vi "導覽&溫度濕度_8月5號.vi"() -> ()   [LabVIEW 2019]
uses:
  Program Files (x86)/National Instruments/LabVIEW 2019/vi.lib/LabVIEW Interface for Arduino/Firmware/LIFA_Base/dht11/DHTXX.lvlib
  <vilib>/LabVIEW Interface for Arduino/LabVIEW Interface for Arduino.lvlib
panel:
  out "?":dbl
  out "濕度(%)":dbl(slide) scale=0.0..100.0
  out "?":dbl
  out "溫度(攝氏)":dbl(knob) scale=0.0..50.0
  in  "開始撥放(影片撥放時，其他作用暫時停用)":bool
  in  "Path":path
  in  "WindowsMediaPlayer":refnum<k7>(container)
  in  "檢測溫度濕度開關":bool
  in  "所有開關停止運作":bool
  out "運作中(燈亮)":bool
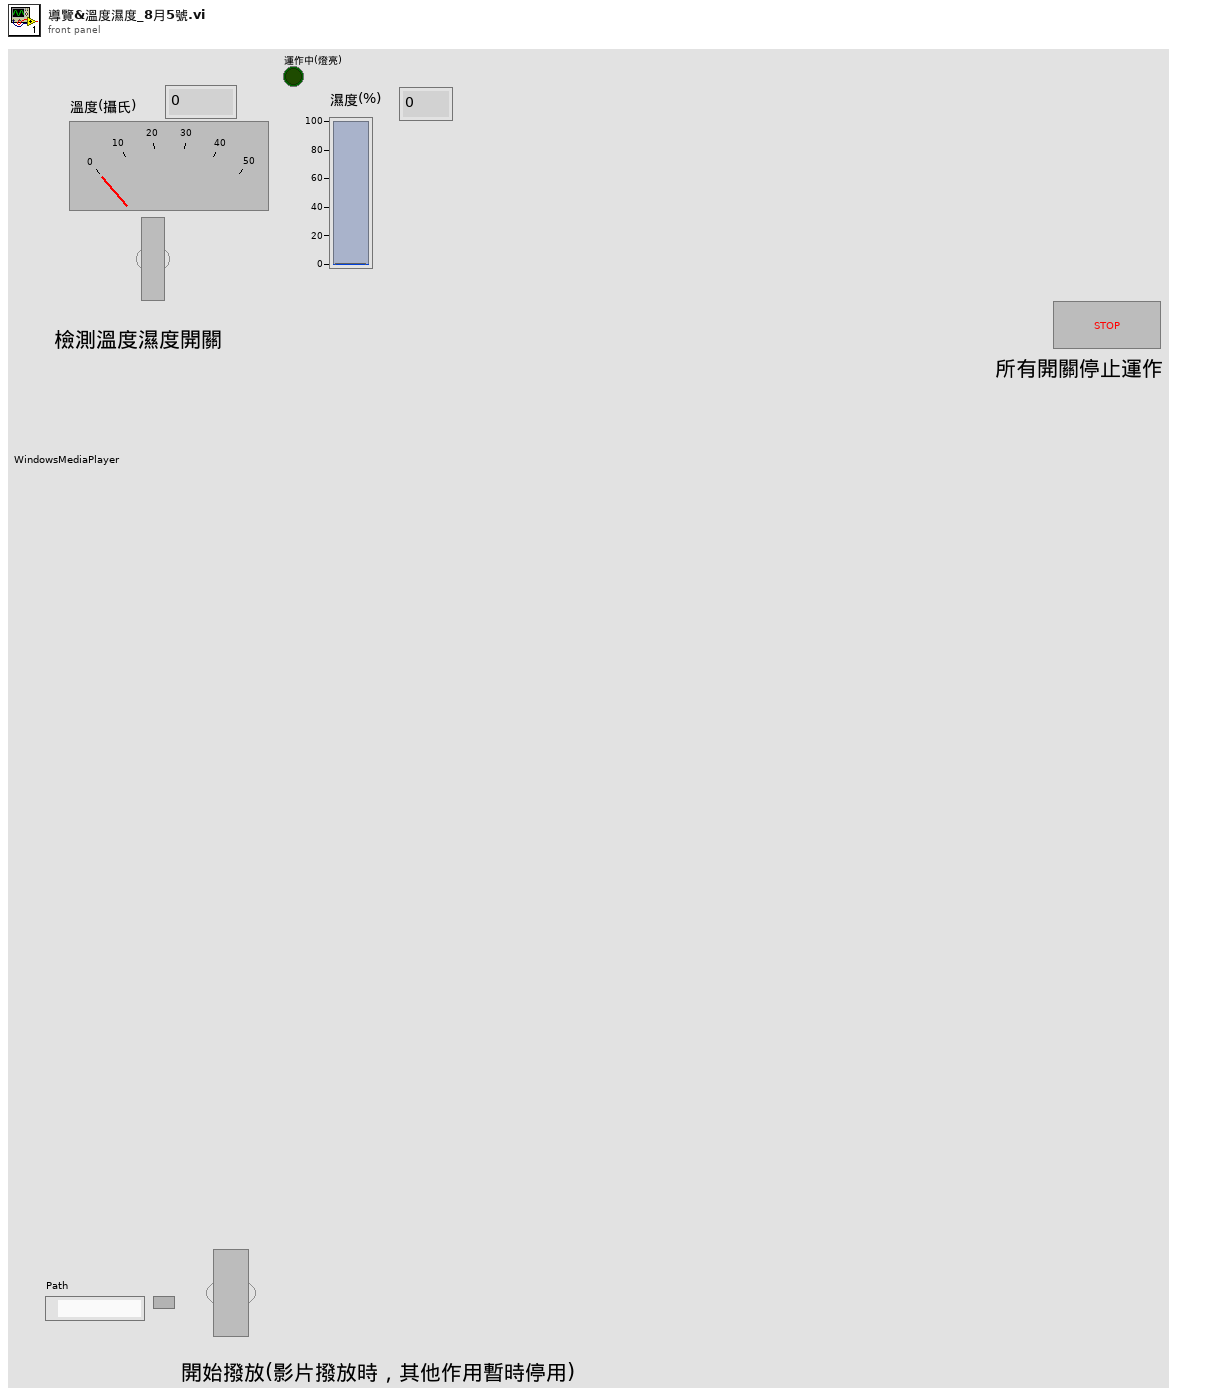
[diagram p1: front panel]
types:
  T1 = typedef "LabVIEW Interface for Arduino.lvlib/Arduino Resource.ctl" = cluster{"VISA resource":refnum<visa-resource-name>, "Board Type":T2, "Connection Type":enum8{"USB / Serial"}, "Bytes Per Packet (15)":u8}
  T2 = typedef "LabVIEW Interface for Arduino.lvlib/Board Type.ctl" = enum16{"Uno", "Dimuelanove w/Atmega 328", "Mega 2560"}
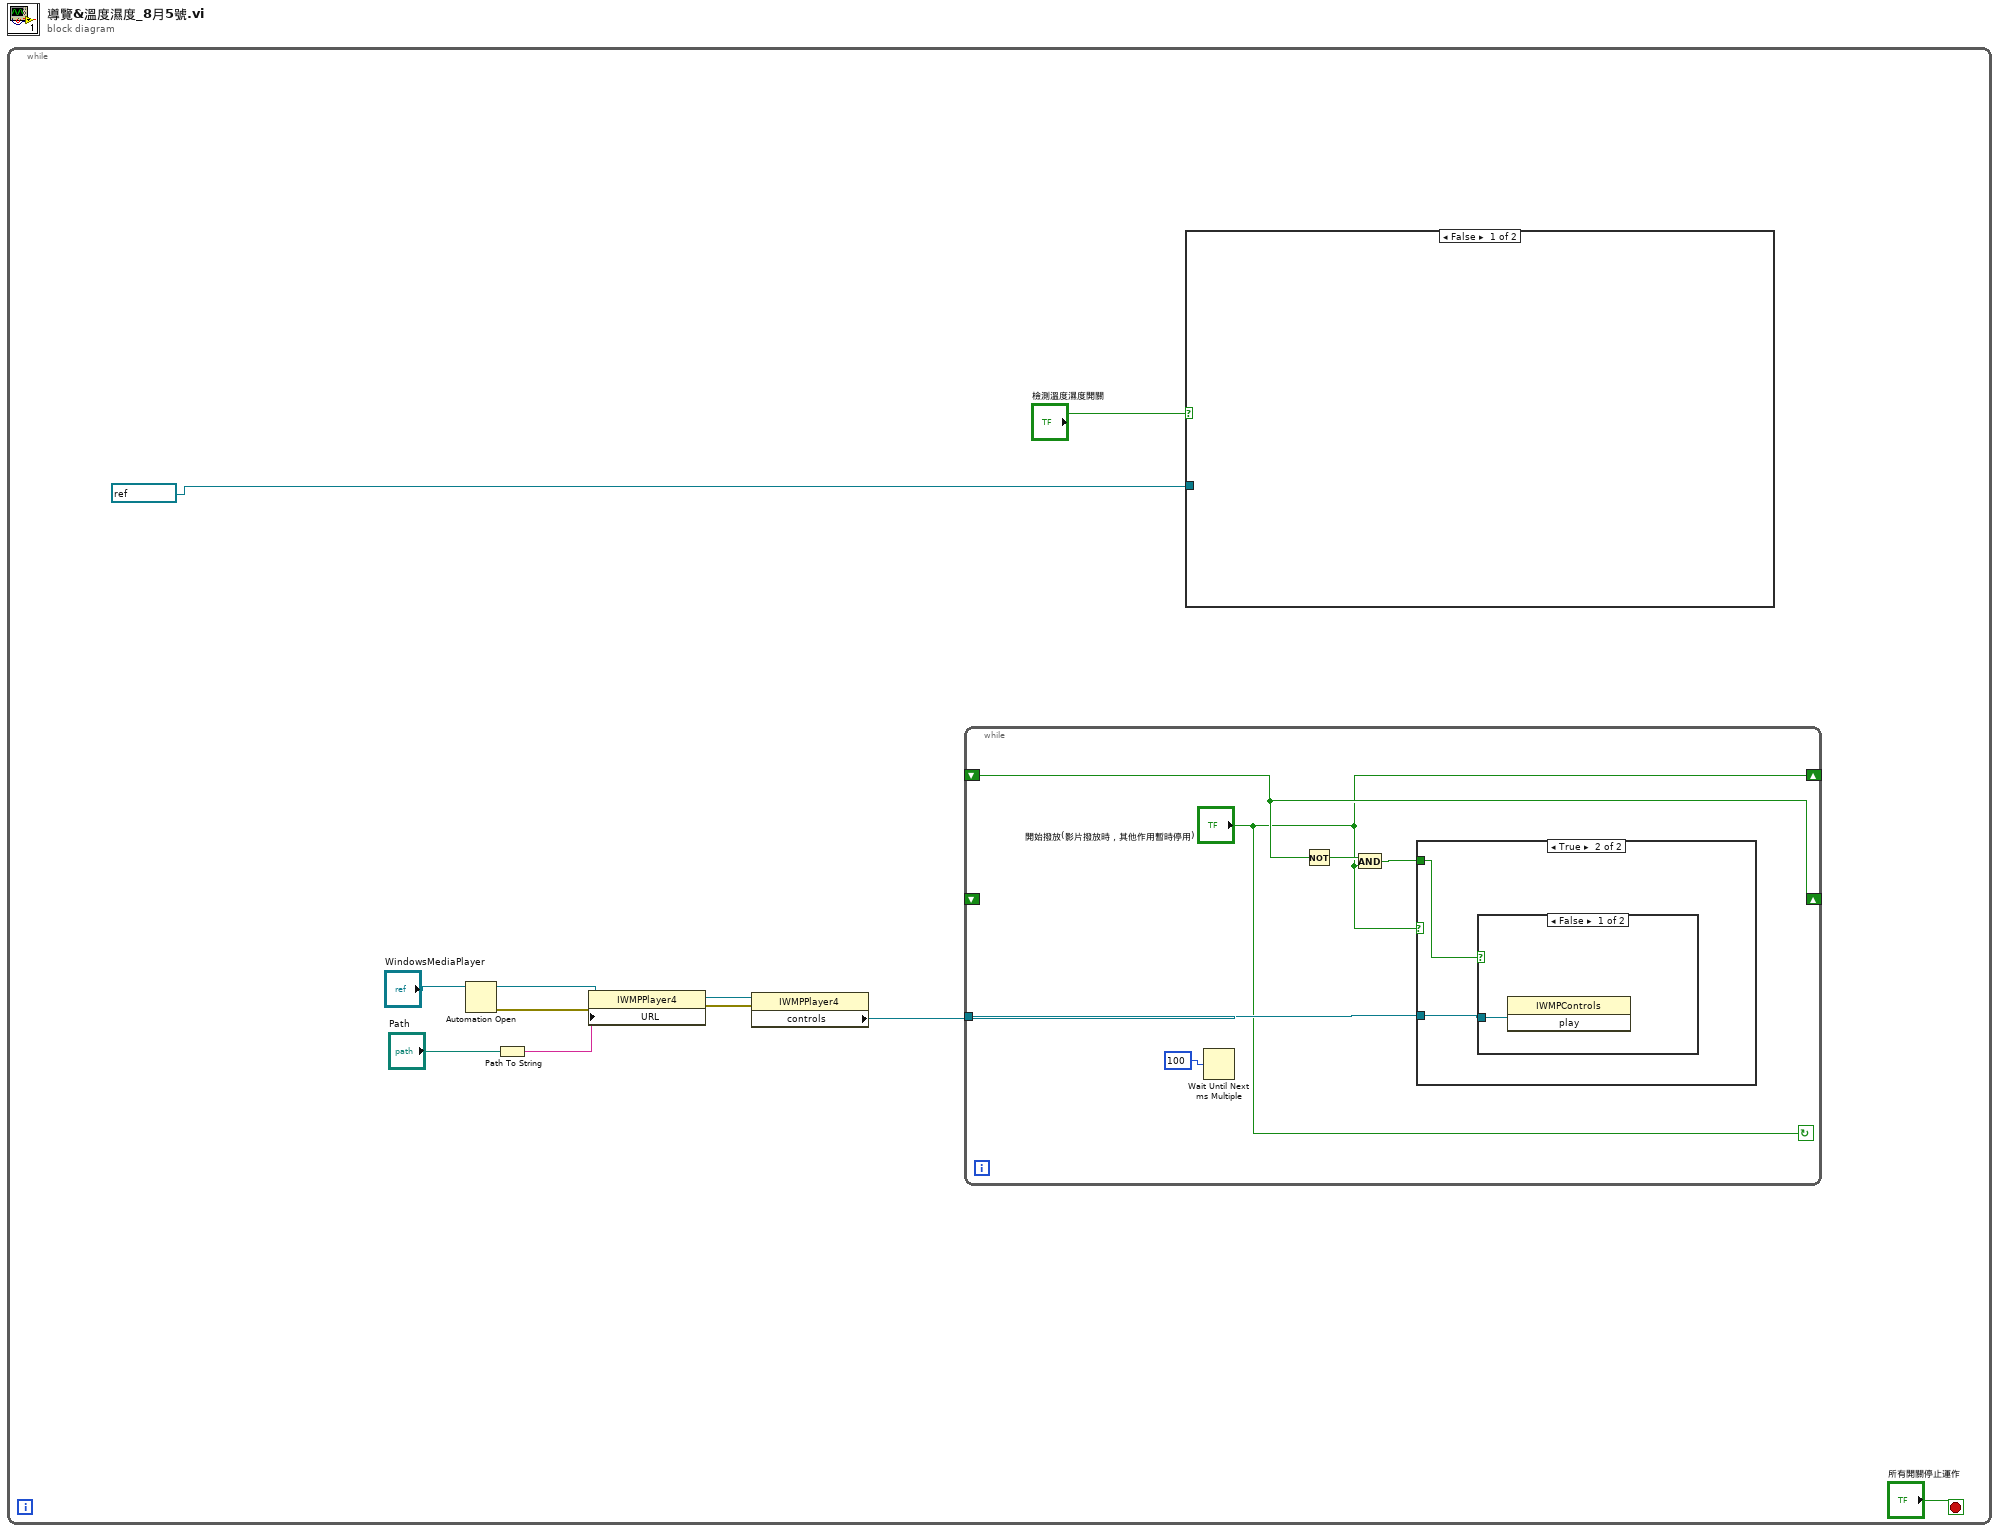
[diagram p0: block diagram]
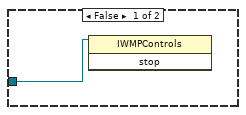
[diagram p2: hidden frame]
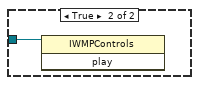
[diagram p3: hidden frame]
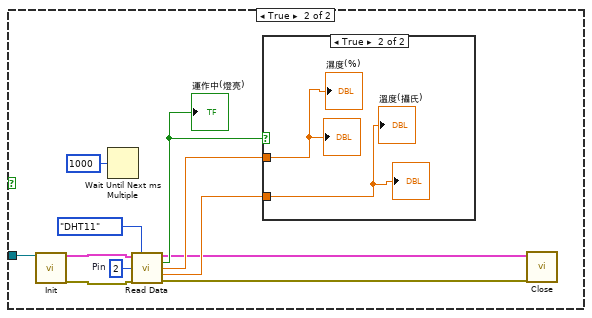
[diagram p4: hidden frame]
diagram:
  n1 = while {
    stop <- "所有開關停止運作" stop-if-true
    n2 = Automation Open(Automation Refnum="WindowsMediaPlayer") -> (Automation Refnum=w3:refnum<k7>, error out=w5:errorcluster)  [unwired: 3 in]
    n3 = Path To String(path="Path") -> (string=w7:string)
    n4 = property class="IWMPPlayer4"(reference=w3, error in=w5, "URL"=w7) -> (reference out=w4:refnum<k7>, error out=w6:errorcluster)
    n5 = property class="IWMPPlayer4"(reference=w4, error in=w6) -> ("controls"=w1:refnum<k7>)  [unwired: 2 out]
    n6 = while {
      tunnel: w1 -> [w17]
      shift-right: [w14] -> _
      shift-left: _ -> [_]
      shift-right: ["開始撥放(影片撥放時，其他作用暫時停用)"] -> _
      shift-left: _ -> [w14]
      stop <- "開始撥放(影片撥放時，其他作用暫時停用)" continue-if-true
      n7 = Wait Until Next ms Multiple(millisecond multiple=u32 100 ("millisecond timer value")) -> ()  [unwired: 1 out]
      n8 = Not(x=w14) -> (.not. x?=w16:bool)
      n9 = And(x=w16, y="開始撥放(影片撥放時，其他作用暫時停用)") -> (x .and. y?=w15:bool)
      n10 = case shown="True" "開始撥放(影片撥放時，其他作用暫時停用)" {
        tunnel: w17 -> [w18 w20]
        tunnel: w15 -> [_ w19]
        frame False {
          n11 = invoke class="IWMPControls" method="stop"(reference=w18) -> ()  [unwired: 2 in, 3 out]
        }
        frame True {
          n12 = case shown="False" w19 {
            tunnel: w20 -> [w21 w22]
            frame False {
              n13 = invoke class="IWMPControls" method="play"(reference=w21) -> ()  [unwired: 2 in, 3 out]
            }
            frame True {
              n14 = invoke class="IWMPControls" method="play"(reference=w22) -> ()  [unwired: 2 in, 3 out]
            }
          }
        }
      }
    }
    n15 = case shown="False" "檢測溫度濕度開關" {
      tunnel: refnum<visa-resource-name> "COM6" ("VISA resource") -> [_ w23]
      frame False {
      }
      frame True {
        w29 = u8 2  # Pin
        n16 = call <vilib>:"Init.vi"("VISA resource"=w23) -> ("Arduino Resource"=w25:T1, "error out"=w24:errorcluster)  [unwired: 17 in]
        n17 = Wait Until Next ms Multiple(millisecond multiple=u32 1000) -> ()  [unwired: 1 out]
        n18 = call "Read Data.vi"("Arduino Resource"=w25, "Sensor Type"=enum16{"DHT11", "DHT21", "DHT22"}."DHT11", "Pin"=w29, "error in (no error)"=w24) -> ("Arduino Resource"=w27:T1, "Successful?"=w33:bool, "Relative Humidity"=w32:dbl, "Temperature (°C)"=w31:dbl, "error out"=w26:errorcluster)  [unwired: 7 in]
        "運作中(燈亮)" <- w33
        n19 = case shown="True" w33 {
          tunnel: w32 -> [_ w34]
          tunnel: w31 -> [_ w35]
          frame False {
          }
          frame True {
            "溫度(攝氏)" <- w35
            "?" <- w35
            "濕度(%)" <- w34
            "?" <- w34
          }
        }
        n20 = call <vilib>:"Close.vi"("Arduino Resource"=w27, "error in"=w26) -> ()  [unwired: 13 in, 1 out]
      }
    }
  }
